vi "CountDiagramsRecursive.vi"(11 "VI in":refnum<vi>) -> (2 "Number of diagrams":i32, 3 "VI out":refnum<vi>)   [LabVIEW 2020]
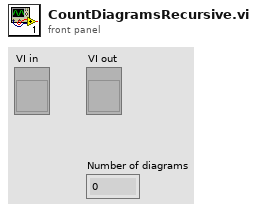
[diagram p1: front panel]
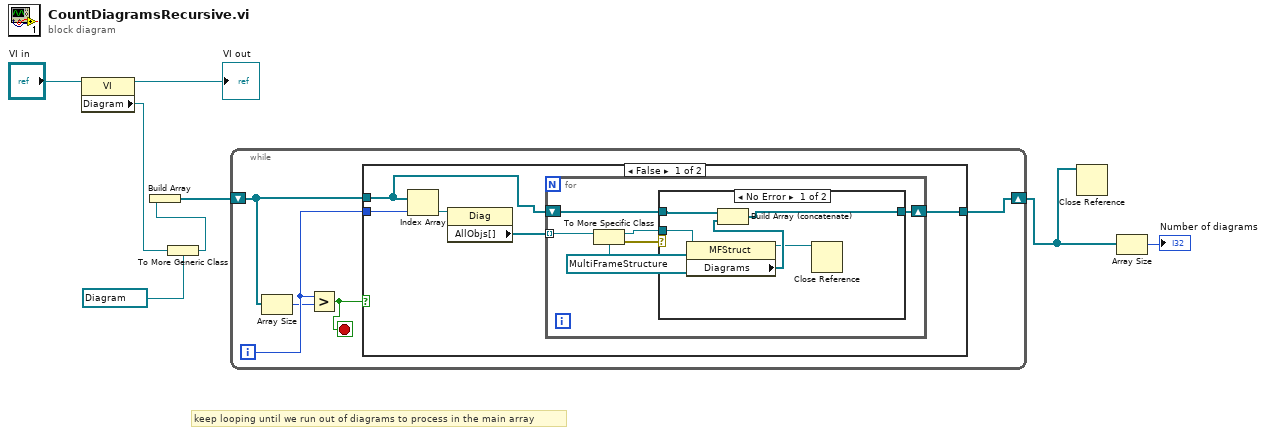
[diagram p0: block diagram]
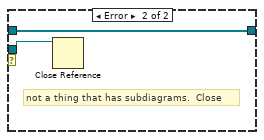
[diagram p2: hidden frame]
diagram:
  # "keep looping until we run out of diagrams to process in the main array"
  n1 = property class="VI"(reference="VI in") -> (reference out=→"VI out":refnum<vi>, "Diagram"=w5:refnum<vi>)  [unwired: 1 in, 1 out]
  n2 = To More Generic Class(target class=refnum<vi> refnum ("Block Diagram"), reference=w5) -> (generic class reference=w4:refnum<vi>)
  n3 = Build Array(w4) -> (w6:refnum<vi>[])
  n4 = while {
    shift-right: [w13] -> w2
    shift-left: w6 -> [w10]
    i -> [w12]
    stop <- w9 stop-if-true
    n5 = Array Size(array=w10) -> (size(s)=w11:i32)
    n6 = Greater?(x=w12, y=w11) -> (0:w9:bool)
    n7 = case shown="False" w9 {
      tunnel: [w16 w32] -> w13
      tunnel: w12 -> [w15 _]
      tunnel: w10 -> [w14 w32]
      frame False {
        n8 = Index Array(array=w14, index=w15) -> (element=w18:refnum<vi>)
        n9 = property class="Diag"(reference=w18) -> ("AllObjs[]"=w17:refnum<vi>[])  [unwired: 1 in, 2 out]
        n10 = for {
          tunnel: w17 -> [w23] mode=indexing
          shift-right: [w19] -> w16
          shift-left: w14 -> [w20]
          n11 = To More Specific Class(target class=refnum<vi> refnum ("Block Diagram"), reference=w23) -> (specific class reference=w21:refnum<vi>, error out=w22:errorcluster)  [unwired: 1 in]
          n12 = case shown="No Error" w22 {
            tunnel: w21 -> [w27 w31]
            tunnel: w20 -> [w29 w30]
            tunnel: [w28 w30] -> w19
            frame No Error {
              n13 = property class="MFStruct"(reference=w27) -> (reference out=w25:refnum<vi>, "Diagrams"=w26:refnum<vi>[])  [unwired: 1 in, 1 out]
              n14 = Build Array (concatenate)(w29, w26) -> (w28:refnum<vi>[])
              n15 = Close Reference(reference=w25) -> ()  [unwired: 1 in, 1 out]
            }
            frame Error {
              # "not a thing that has subdiagrams.  Close"
              n16 = Close Reference(reference=w31) -> ()  [unwired: 1 in, 1 out]
            }
          }
        }
      }
      frame True {
        # "Nothing left to do"
      }
    }
  }
  n17 = Close Reference(reference=w2) -> ()  [unwired: 1 in, 1 out]
  n18 = Array Size(array=w2) -> (size(s)=→"Number of diagrams":i32)
